vi "FPGAPackets.vi"(0 "Repeats":u32=1, 1 "Period (ns)":dbl=5.0, 2 "Durations":dbl[](array[numeric]), 3 "States":string[](array[string]), 4 "Trigger":bool) -> (5 "Packets":string, 6 "Bytes":u8[](array[numeric]))   [LabVIEW 2014]
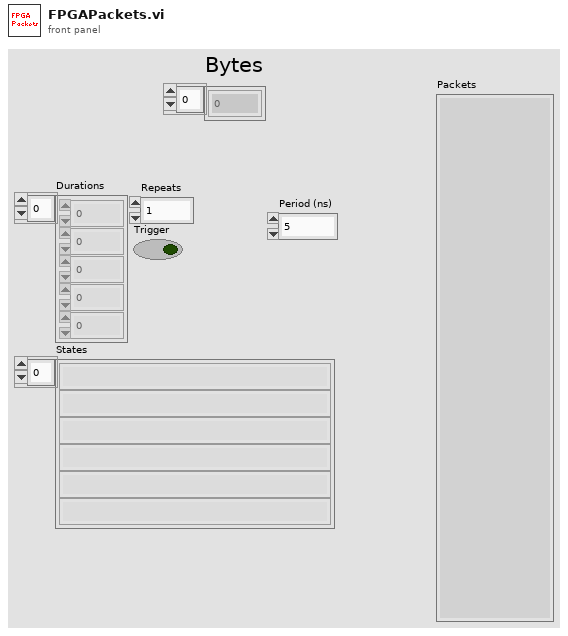
[diagram p1: front panel]
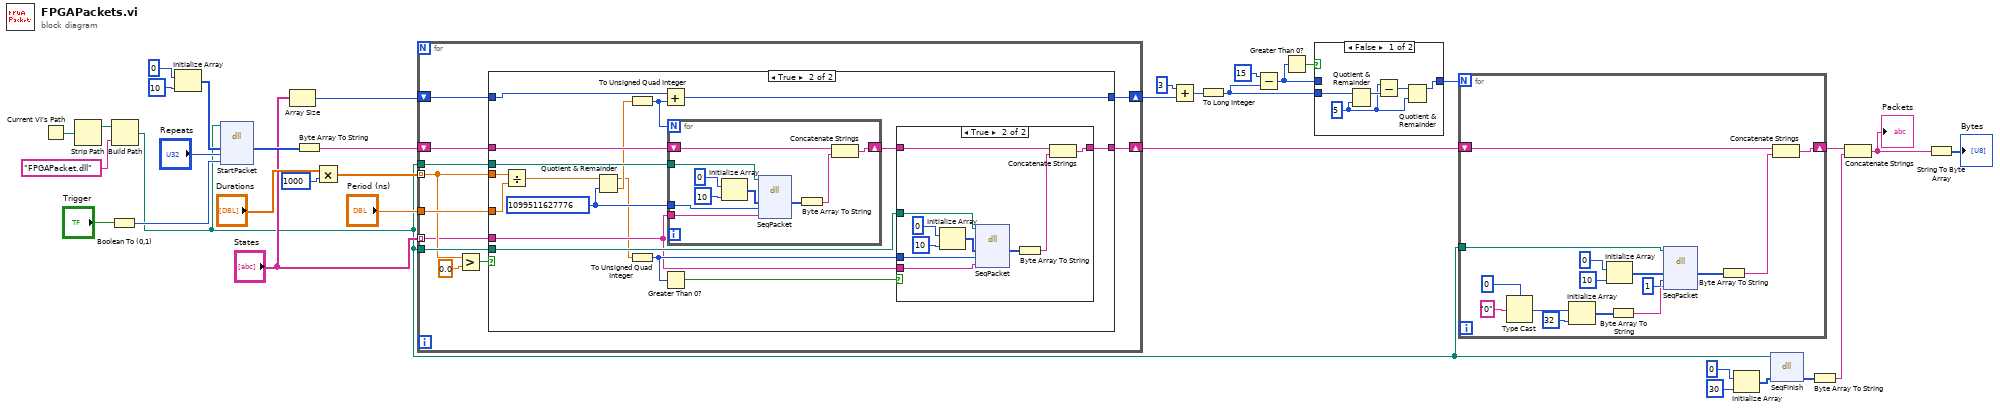
[diagram p0: block diagram]
diagram:
  n1 = Current VI's Path() -> (path=w4:path)
  n2 = Strip Path(path=w4) -> (stripped path=w3:path)  [unwired: 1 out]
  n3 = Boolean To (0,1)(Boolean="Trigger") -> (0, 1=w8:i16)
  n4 = Build Path(base path=w3, name or relative path="FPGAPacket.dll") -> (appended path=w1:path)
  n5 = Initialize Array(u8 0 ("element"), 10 ("dimension size")) -> (w33:u8[])
  n6 = dll-call lib="D:/Desktop/LabVIEW/Sequencer/FPGAPacket.dll" fn="StartPacket"(path in=w1, "packet"=w33, "repeats"="Repeats", "trigger"=w8) -> ("packet"=w32:u8[])  [unwired: 5 in, 2 out]
  n7 = Array Size(array="States") -> (size(s)=w12:i32)
  n8 = Byte Array To String(unsigned byte array=w32) -> (string=w14:string)
  n9 = Multiply(x="Durations", y=1000) -> (x*y=w21:dbl[])
  n10 = for {
    tunnel: "States" -> [w36] mode=indexing
    tunnel: w21 -> [w38] mode=indexing
    tunnel: "Period (ns)" -> [w46]
    shift-right: [w45] -> w30
    shift-left: w14 -> [w43]
    tunnel: w1 -> [w44]
    tunnel: w1 -> [w42]
    shift-right: [w40] -> w11
    shift-left: w12 -> [w41]
    n11 = Greater?(x=w38, y=0.0) -> (0:w37:bool)
    n12 = case shown="True" w37 {
      tunnel: w38 -> [_ w65]
      tunnel: w46 -> [_ w64]
      tunnel: [w48 w63] -> w45
      tunnel: w44 -> [_ w62]
      tunnel: w43 -> [w48 w60]
      tunnel: w42 -> [_ w57]
      tunnel: w41 -> [w47 w56]
      tunnel: [w47 w55] -> w40
      tunnel: w36 -> [_ w51]
      frame False {
      }
      frame True {
        w58 = u64 1099511627776 ("y")
        n13 = Divide(x=w65, y=w64) -> (x/y=w61:dbl)
        n14 = Quotient & Remainder(x=w61, y=w58) -> (x-y*floor(x/y)=w49:dbl, floor(x/y)=w50:dbl)
        n15 = To Unsigned Quad Integer(1:w50) -> (0:w54:u64)
        n16 = To Unsigned Quad Integer(1:w49) -> (0:w52:u64)
        n17 = Add(x=w56, y=w54) -> (x+y=w55:u64)
        n18 = Greater Than 0?(x=w52) -> (x > 0?=w53:bool)
        n19 = for {
          N: w54 -> [_]
          shift-right: [w78] -> w59
          shift-left: w60 -> [w79]
          tunnel: w58 -> [w86]
          tunnel: w51 -> [w82]
          tunnel: w57 -> [w77]
          n20 = Initialize Array(u8 0 ("element"), 10 ("dimension size")) -> (w84:u8[])
          n21 = dll-call lib="D:/Desktop/LabVIEW/Sequencer/FPGAPacket.dll" fn="SeqPacket"(path in=w77, "packet"=w84, "duration"=w86, "state"=w82) -> ("packet"=w81:u8[])  [unwired: 5 in, 2 out]
          n22 = Byte Array To String(unsigned byte array=w81) -> (string=w80:string)
          n23 = Concatenate Strings(w79, w80) -> (w78:string)
        }
        n24 = case shown="True" w53 {
          tunnel: [w66 w71] -> w63
          tunnel: w62 -> [_ w70]
          tunnel: w52 -> [_ w69]
          tunnel: w59 -> [w66 w68]
          tunnel: w51 -> [_ w67]
          frame False {
          }
          frame True {
            n25 = Initialize Array(u8 0 ("element"), 10 ("dimension size")) -> (w73:u8[])
            n26 = dll-call lib="D:/Desktop/LabVIEW/Sequencer/FPGAPacket.dll" fn="SeqPacket"(path in=w70, "packet"=w73, "duration"=w69, "state"=w67) -> ("packet"=w76:u8[])  [unwired: 5 in, 2 out]
            n27 = Byte Array To String(unsigned byte array=w76) -> (string=w72:string)
            n28 = Concatenate Strings(w68, w72) -> (w71:string)
          }
        }
      }
    }
  }
  n29 = Add(x=3, y=w11) -> (x+y=w10:u64)
  n30 = To Long Integer(number=w10) -> (32bit integer=w9:i32)
  n31 = Subtract(x=15, y=w9) -> (x-y=w16:i32)
  n32 = Greater Than 0?(x=w16) -> (x > 0?=w19:bool)
  n33 = case shown="False" w19 {
    tunnel: w16 -> [_ w92]
    tunnel: [w87 w92] -> w15
    tunnel: w9 -> [w88 _]
    frame False {
      w89 = u32 5 ("y")
      n34 = Quotient & Remainder(x=w88, y=w89) -> (x-y*floor(x/y)=w91:u32)  [unwired: 1 out]
      n35 = Subtract(x=w89, y=w91) -> (x-y=w90:u32)
      n36 = Quotient & Remainder(x=w90, y=w89) -> (x-y*floor(x/y)=w87:u32)  [unwired: 1 out]
    }
    frame True {
    }
  }
  n37 = for {
    N: w15 -> [_]
    shift-right: [w96] -> w25
    shift-left: w30 -> [w95]
    tunnel: w1 -> [w93]
    n38 = Type Cast(type=u8 0 ("element"), x="0") -> (*(type *) &x=w99:u8)
    n39 = Initialize Array(w99, 32 ("dimension size")) -> (w102:u8[])
    n40 = Initialize Array(u8 0 ("element"), 10 ("dimension size")) -> (w105:u8[])
    n41 = Byte Array To String(unsigned byte array=w102) -> (string=w101:string)
    n42 = dll-call lib="D:/Desktop/LabVIEW/Sequencer/FPGAPacket.dll" fn="SeqPacket"(path in=w93, "packet"=w105, "duration"=u64 1, "state"=w101) -> ("packet"=w97:u8[])  [unwired: 5 in, 2 out]
    n43 = Byte Array To String(unsigned byte array=w97) -> (string=w94:string)
    n44 = Concatenate Strings(w95, w94) -> (w96:string)
  }
  n45 = Initialize Array(u8 0 ("element"), 30 ("dimension size")) -> (w27:u8[])
  n46 = dll-call lib="D:/Desktop/LabVIEW/Sequencer/FPGAPacket.dll" fn="SeqFinish"(path in=w1, "packet"=w27) -> ("packet"=w26:u8[])  [unwired: 3 in, 2 out]
  n47 = Byte Array To String(unsigned byte array=w26) -> (string=w24:string)
  n48 = Concatenate Strings(w25, w24) -> (w6:string)
  "Packets" <- w6
  n49 = String To Byte Array(string=w6) -> (unsigned byte array=→"Bytes":u8[])
